vi "ZBCgate.vi"() -> ()   [LabVIEW 2010]
panel:
  in  "Integration Time(ms)":dbl
  out "Data Points":dbl
  out "Sweep Time (s)":dbl
  out "XY Graph":cluster{"Y":dbl[], "Y":dbl[]}[](graph)
  in  "Channel":u16(ring)
  in  "End Settling Time(ms)":dbl
  in  "Settling Time(ms)":dbl
  in  "Increment Gate (V)":dbl
  in  "Initial Settling Time(ms)":dbl
  in  "End Gate (V)":dbl
  in  "Start Gate (V)":dbl
  in  "File name":string
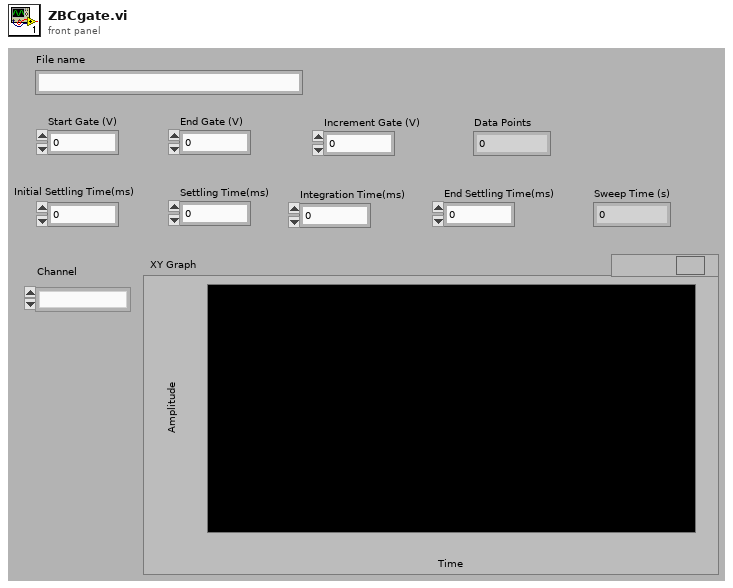
[diagram p1: front panel]
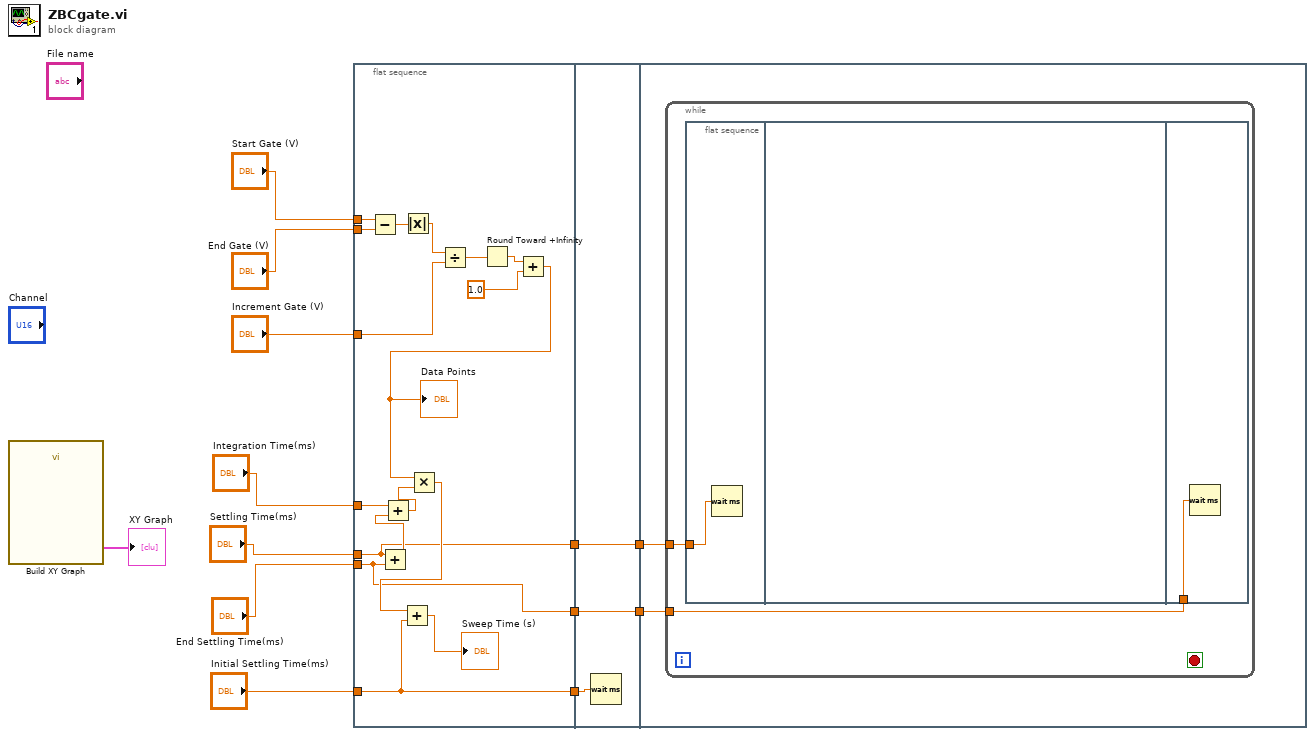
[diagram p0: block diagram]
diagram:
  n1 = call "Build XY Graph"() -> ("XY Graph"=→"XY Graph":cluster{"Y":dbl[], "Y":dbl[]}[])  [unwired: 5 in, 6 out]
  n2 = flat-sequence {
    tunnel: "Start Gate (V)" -> [w30]
    tunnel: "End Gate (V)" -> [w29]
    tunnel: "Increment Gate (V)" -> [w27]
    tunnel: "Settling Time(ms)" -> [w15]
    tunnel: "End Settling Time(ms)" -> [w14]
    tunnel: "Initial Settling Time(ms)" -> [w19]
    tunnel: [w19] -> w6
    tunnel: "Integration Time(ms)" -> [w16]
    tunnel: [w15] -> w4
    tunnel: [w14] -> w2
    tunnel: w6 -> [w33]
    tunnel: w4 -> [w32]
    tunnel: [w32] -> w3
    tunnel: w2 -> [w31]
    tunnel: [w31] -> w1
    tunnel: w3 -> [w35]
    tunnel: w1 -> [w34]
    frame #0 {
      n3 = Subtract(x=w30, y=w29) -> (x-y=w28:dbl)
      n4 = Add(x=w15, y=w14) -> (x+y=w17:dbl)
      n5 = Add(x=w16, y=w17) -> (x+y=w18:dbl)
      n6 = Absolute Value(x=w28) -> (abs(x)=w26:dbl)
      n7 = Divide(x=w26, y=w27) -> (x/y=w25:dbl)
      n8 = Round Toward +Infinity(x=w25) -> (ceil(x): smallest int >= x=w24:dbl)
      n9 = Add(x=w24, y=1.0) -> (x+y=w22:dbl)
      "Data Points" <- w22
      n10 = Multiply(x=w22, y=w18) -> (x*y=w21:dbl)
      n11 = Add(x=w21, y=w19) -> (x+y=→"Sweep Time (s)":dbl)
    }
    frame #1 {
      n12 = Wait (ms)(milliseconds to wait=w33) -> ()  [unwired: 1 out]
    }
    frame #2 {
      n13 = while {
        tunnel: w35 -> [w37]
        tunnel: w34 -> [w36]
        stop <- _ stop-if-true
        n14 = flat-sequence {
          tunnel: w37 -> [w38]
          tunnel: w36 -> [w39]
          frame #0 {
            n15 = Wait (ms)(milliseconds to wait=w38) -> ()  [unwired: 1 out]
          }
          frame #1 {
          }
          frame #2 {
            n16 = Wait (ms)(milliseconds to wait=w39) -> ()  [unwired: 1 out]
          }
        }
      }
    }
  }
